vi "Set Value.vi"(8 "error in (no error)":errorcluster, 10 "Value":variant, 11 "String Type View in":refnum<class "Integer Type View.lvclass">) -> (0 "error out":errorcluster, 3 "String Type View out":refnum<class "Integer Type View.lvclass">)   [LabVIEW 2017, in "Integer Type View.lvclass"]
uses:
  <vilib>/gpm_packages/@cs/Test-executive-builder/Source/Test Executive Builder Dialogs/Integer Type View/Integer Type View.lvclass
  <vilib>/gpm_packages/@cs/Test-executive-builder/Source/Test Executive Builder Dialogs/Integer Type View/Integer Type View.lvclass/Integer Type View.ctl
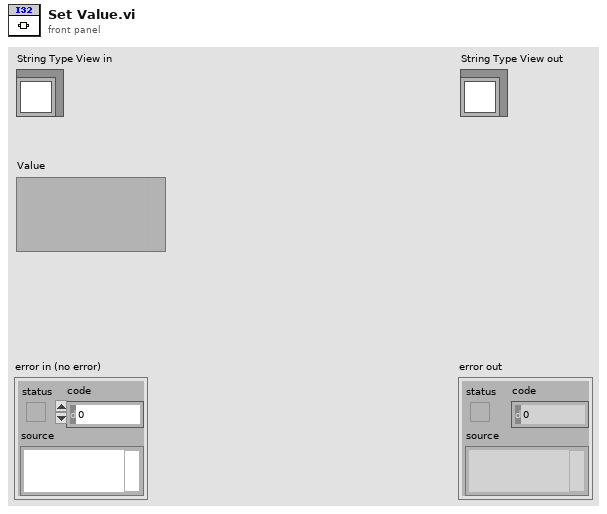
[diagram p1: front panel]
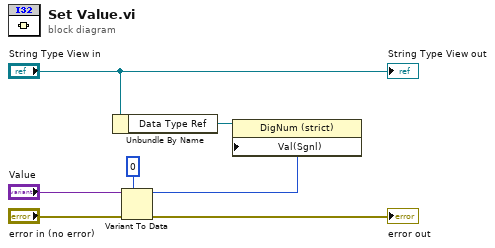
[diagram p0: block diagram]
diagram:
  n1 = Unbundle By Name("String Type View in") -> ("Data Type Ref"=w3:refnum<vi>)
  n2 = Variant To Data(error in="error in (no error)", type=0, Variant="Value") -> (data=w1:i32, error out=→"error out":errorcluster)
  n3 = property class="DigNum (strict)"(reference=w3, "Val(Sgnl)"=w1) -> ()  [unwired: 1 in, 2 out]
  "String Type View out" <- "String Type View in"
